vi "Func_Glob_TriAndTree_PN.vi"(2 "Trimmed down TreeNode array IN":T1[](array[typedef]), 3 "Corrected triangles IN":T2[](array[typedef]), 4 "Action":enum16{"Read", "Write"}(ring)) -> (0 "Trimmed down TreeNode array OUT":T1[](array[typedef]), 1 "Corrected triangles OUT":T2[](array[typedef]))   [LabVIEW 2010]
uses:
  Triangle2D.ctl
  Qtree vis/Trimmed down TreeNode2D.ctl
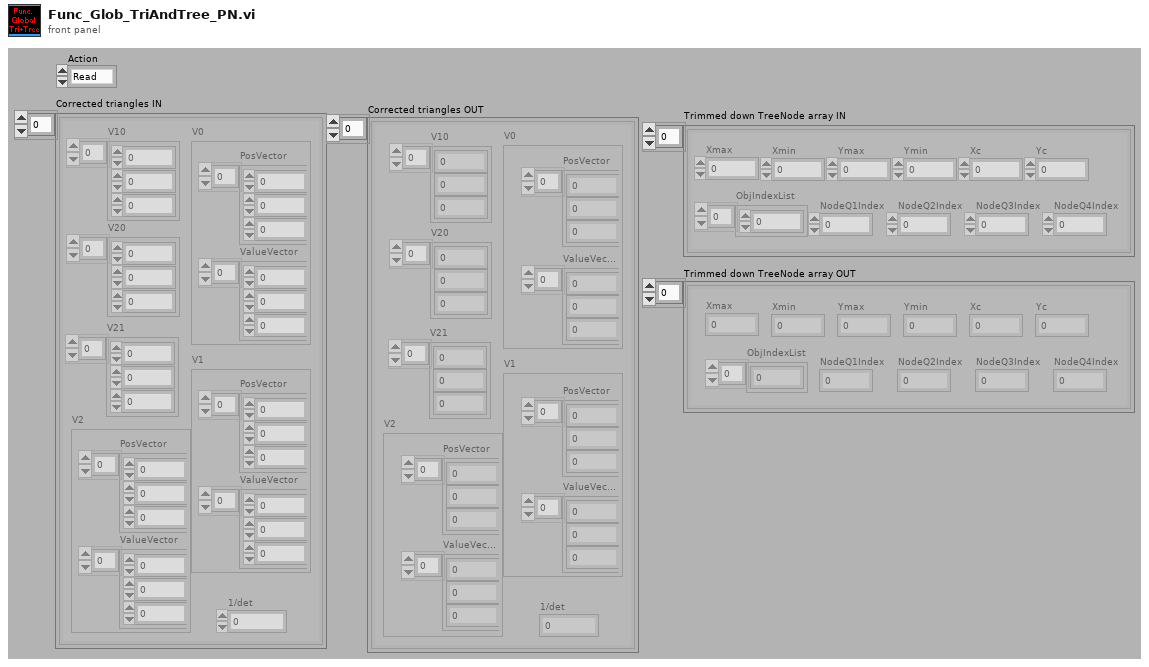
[diagram p1: front panel]
types:
  T1 = typedef "Trimmed down TreeNode2D.ctl" = cluster{"Xmax":dbl, "Xmin":dbl, "Ymax":dbl, "Ymin":dbl, "Xc":dbl, "Yc":dbl, "ObjIndexList":i32[], "NodeQ1Index":i32, "NodeQ2Index":i32, "NodeQ3Index":i32, "NodeQ4Index":i32}
  T2 = typedef "Triangle2D.ctl" = cluster{"V10":dbl[], "V20":dbl[], "1/det":dbl, "V0":cluster{"PosVector":dbl[], "ValueVector":dbl[]}, "V1":cluster{"PosVector":dbl[], "ValueVector":dbl[]}, "V2":cluster{"PosVector":dbl[], "ValueVector":dbl[]}, "V21":dbl[]}
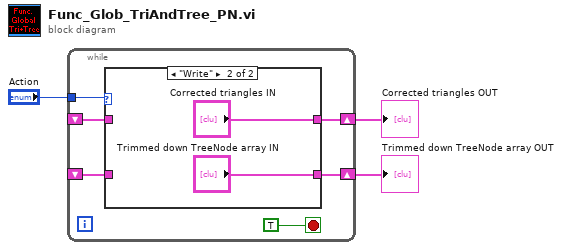
[diagram p0: block diagram]
diagram:
  n1 = while {
    shift-right: [w5] -> w2
    shift-left: _ -> [w7]
    shift-right: [w4] -> w1
    shift-left: _ -> [w6]
    tunnel: "Action" -> [w9]
    stop <- TRUE stop-if-true
    n2 = case shown="\"Write\"" w9 {
      tunnel: w7 -> [w11 _]
      tunnel: w6 -> [w10 _]
      tunnel: [w11 "Corrected triangles IN"] -> w5
      tunnel: [w10 "Trimmed down TreeNode array IN"] -> w4
      frame "Read" {
      }
      frame "Write" {
      }
    }
  }
  "Corrected triangles OUT" <- w2
  "Trimmed down TreeNode array OUT" <- w1
